vi "Change Laser Off Time.vi"(8 "error in":errorcluster, 11 "tCRD in":refnum<class "Open Path CRD.lvclass">) -> (0 "error out":errorcluster, 3 "tCRD out":refnum<class "Open Path CRD.lvclass">)   [LabVIEW 2015, in "Open Path CRD.lvclass"]
uses:
  Open Path CRD.lvclass
  Reusable/Instrument/Instrument.lvclass/Instrument.ctl
  Open Path CRD.lvclass/Open Path CRD.ctl
  Reusable/Instrument/Read Log Session.vi
  Accessors/Read FPGA Ref.vi
  Reusable/Instrument/Write Restart Requested_.vi
  <vilib>/Utility/error.llb/Error Cluster From Error Code.vi
  <vilib>/rvi/errors/niLvFpgaAdjustHostInterfaceError.vi
  <userlib>/_Session Fwk/Session - Root.lvclass
  <vilib>/rvi/interface/nirviReadWriteControl/nirviReadWriteControl.xnode
  Open Path FPGA Ref.ctl
  FPGA Bitfiles/Handix_OpenPathCRD.lvbitx
  Reusable/Session Log/System Log.lvclass
  Reusable/Instrument/Instrument.lvclass
  NiFpgaLv.dll
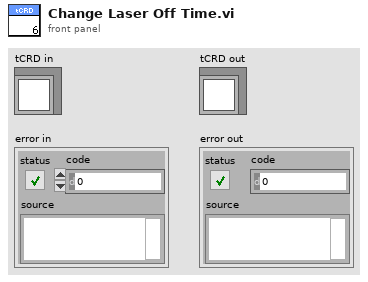
[diagram p1: front panel]
types:
  T1 = typedef "Session - Root.lvclass/Session Handle.ctl" = refnum<data-value>
  T2 = typedef "tCRD.lvclass/tFPGA Ref.ctl" = refnum<k20>
  T3 = typedef "Open Path CRD.lvclass/Open Path FPGA Ref.ctl" = refnum<k20>
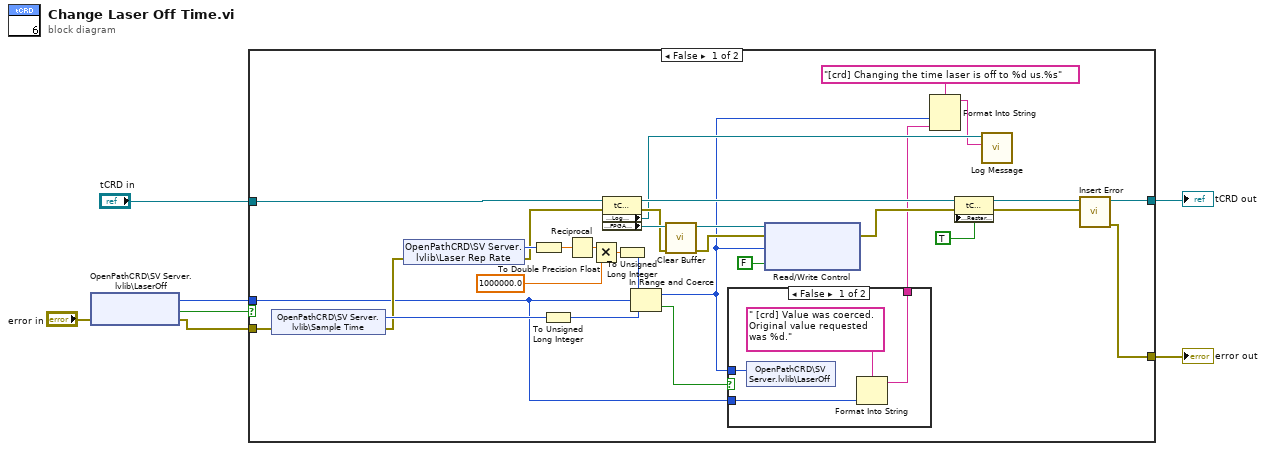
[diagram p0: block diagram]
diagram:
  n1 = shared-variable "OpenPathCRD\\SV Server.lvlib\\LaserOff"(error in="error in") -> (w7:u32, error out=w5:errorcluster, w1:bool)  [unwired: 1 in]
  n2 = case shown="False" w1 {
    tunnel: w7 -> [w14 _]
    tunnel: "tCRD in" -> [w38 w44]
    tunnel: [w9 w44] -> w3
    tunnel: w5 -> [w19 w43]
    tunnel: [w8 w43] -> w4
    frame False {
      n3 = shared-variable "OpenPathCRD\\SV Server.lvlib\\Sample Time"(error in=w19) -> (w24:u16, error out=w18:errorcluster)
      n4 = shared-variable "OpenPathCRD\\SV Server.lvlib\\Laser Rep Rate"(error in=w18) -> (w34:u16, error out=w17:errorcluster)
      n5 = To Double Precision Float(number=w34) -> (double precision float=w33:dbl)
      n6 = To Unsigned Long Integer(number=w24) -> (unsigned 32bit integer=w35:u32)
      n7 = Reciprocal(x=w33) -> (1/x=w37:dbl)
      n8 = Multiply(x=w37, y=1000000.0) -> (x*y=w32:dbl)
      n9 = property class="tCRD"(reference=w38, error in=w17) -> (reference out=w27:refnum<class "Open Path CRD.lvclass">, error out=w22:errorcluster, "Accessors:Log Session"=w20:T1, "Accessors:FPGA Ref"=w23:T2)
      n10 = To Unsigned Long Integer(number=w32) -> (unsigned 32bit integer=w31:u32)
      n11 = In Range and Coerce(upper limit=w31, x=w14, lower limit=w35) -> (coerced(x)=w15:u32, In Range?=w30:bool)
      n12 = call "Clear Buffer.vi"("error in"=w22, "Refnum in"=w23) -> ("error out"=w21:errorcluster, "FPGA VI Reference Out"=w29:T3)  [unwired: 8 in]
      n13 = case shown="False" w30 {
        tunnel: w15 -> [w42 _]
        tunnel: w14 -> [w40 _]
        tunnel: [w39 _] -> w13
        frame False {
          n14 = shared-variable "OpenPathCRD\\SV Server.lvlib\\LaserOff"(w42) -> ()  [unwired: 1 in, 1 out]
          n15 = Format Into String(format string=" [crd] Value was coerced.  Original value requested was %d.", w40) -> (resulting string=w39:string)  [unwired: 2 in, 1 out]
        }
        frame True {
        }
      }
      n16 = xnode "Read/Write Control"("FPGA VI Reference In"=w29, "error in"=w21, "LaserOff (us)"=w15, "Pause Digitizer"=FALSE) -> ("error out"=w26:errorcluster)  [unwired: 1 out]
      n17 = Format Into String(format string="[crd] Changing the time laser is off to %d us.%s", w15, w13) -> (resulting string=w12:string)  [unwired: 2 in, 1 out]
      n18 = property class="tCRD"(reference=w27, error in=w26, "Accessors:Restart Requested_"=TRUE ("Restart Requested_")) -> (reference out=w11:refnum<class "Open Path CRD.lvclass">, error out=w10:errorcluster)
      n19 = call "Log Message.vi"("MSG In"=w12, "session in"=w20) -> ()  [unwired: 8 in, 2 out]
      n20 = call "Insert Error.vi"("err"=w10, "Instrument in"=w11) -> ("error out"=w8:errorcluster, "Instrument out"=w9:refnum<class "Open Path CRD.lvclass">)  [unwired: 7 in, 1 out]
    }
    frame True {
    }
  }
  "error out" <- w4
  "tCRD out" <- w3
